vi "PreSequenceAcquisition.vi"(8 "error in (no error)":errorcluster, 11 "Camera_Prime95B in":refnum<class "Camera_Prime95B.lvclass">) -> (0 "error out":errorcluster, 3 "Camera_Prime95B out":refnum<class "Camera_Prime95B.lvclass">)   [LabVIEW 2020, in "Camera_Prime95B.lvlib" / "Camera_Prime95B.lvclass"]
uses:
  Camera_Prime95B.lvclass
  Hardware Abstraction Layer/Component/Device/Device/DataExchange.ctl
  Controls/AcquisitionParams.ctl
  Camera_Prime95B.lvclass/Camera_Prime95B.ctl
  E:/Development/DevHardSoftware/MicroscopyFramework/Model/Hardware Layer/Real Hardware/Camera_Prime95B/Camera_Prime95B/Dependencies/PVCamNET.dll
  Dependencies/PVCamNET.dll
  Interface/DataListener/DataListener.lvclass
panel:
  in  "DataExchange":T1
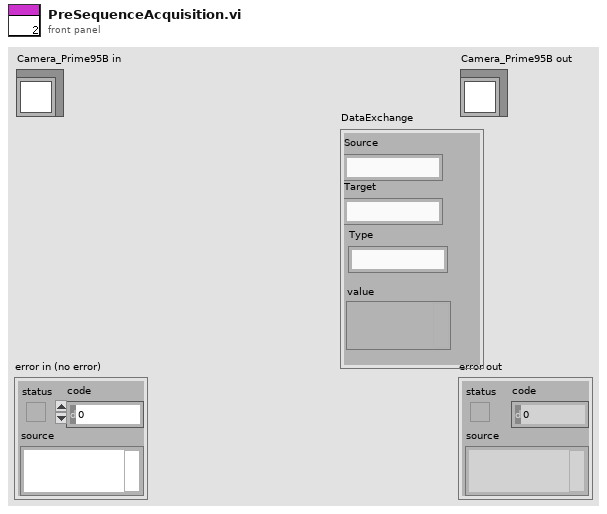
[diagram p1: front panel]
types:
  T1 = typedef "DataListener.lvclass/DataExchange.ctl" = cluster{"Source":string, "Target":string, "Type":string, "value":variant}
  T2 = typedef "Camera_Prime95B.lvlib/Camera_Prime95B.lvclass/AcquisitionParams.ctl" = cluster{"ExposureMs":dbl, "Frames":dbl, "Interval":dbl, "Save Path":path, "Stream Save Path":path, "SingleStack?":bool, "StreamToDisk?":bool, "Alert when finish?":bool, "File suffix":string, "Live?":bool}
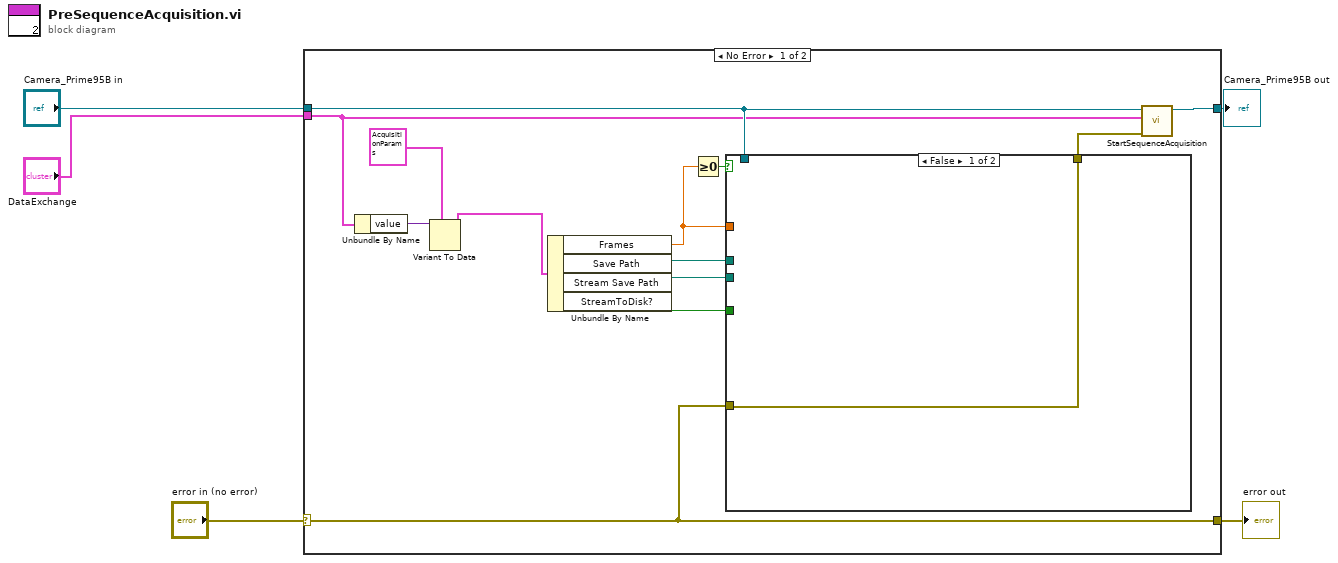
[diagram p0: block diagram]
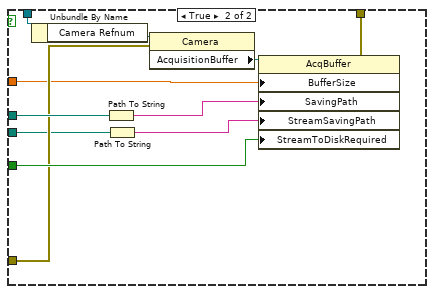
[diagram p2: hidden frame]
diagram:
  n1 = case shown="No Error" "error in (no error)" {
    selector: "error in (no error)" -> [w13 w32]
    tunnel: [w13 w32] -> w4
    tunnel: [w18 w31] -> w2
    tunnel: "Camera_Prime95B in" -> [w15 w31]
    tunnel: "DataExchange" -> [w8 _]
    frame No Error {
      n2 = Unbundle By Name(w8) -> ("value"=w9:variant)
      n3 = Variant To Data(type=T2 {"ExposureMs"=0.0, "Frames"=0.0, "Interval"=0.0, "Save Path"=path "", "Stream Save Path"=path "", "SingleStack?"=FALSE, "StreamToDisk?"=FALSE, "Alert when finish?"=FALSE, "File suffix"="", "Live?"=FALSE} ("Acquisition Params"), Variant=w9) -> (data=w7:T2)  [unwired: 1 in, 1 out]
      n4 = Unbundle By Name(w7) -> ("Frames"=w10:dbl, "Save Path"=w16:path, "Stream Save Path"=w11:path, "StreamToDisk?"=w12:bool)
      n5 = Greater Or Equal To 0?(x=w10) -> (x >= 0?=w17:bool)
      n6 = case shown="False" w17 {
        tunnel: w16 -> [_ w26]
        tunnel: w15 -> [_ w30]
        tunnel: w12 -> [_ w27]
        tunnel: [w19 w25] -> w14
        tunnel: w13 -> [w19 w24]
        tunnel: w11 -> [_ w23]
        tunnel: w10 -> [_ w20]
        frame False {
        }
        frame True {
          n7 = Unbundle By Name(w30) -> ("Camera Refnum"=w29:refnum<k24>)
          n8 = Path To String(path=w26) -> (string=w21:string)
          n9 = Path To String(path=w23) -> (string=w22:string)
          n10 = property class="Camera"(reference=w29, error in=w24) -> ("AcquisitionBuffer"=w28:refnum<k24>)  [unwired: 2 out]
          n11 = property class="AcqBuffer"(reference=w28, "BufferSize"=w20, "SavingPath"=w21, "StreamSavingPath"=w22, "StreamToDiskRequired"=w27) -> (error out=w25:errorcluster)  [unwired: 1 in, 1 out]
        }
      }
      n12 = call-dynamic "StartSequenceAcquisition.vi"("error in (no error)"=w14, "DataExchange"=w8, "Camera_Prime95B in"=w15) -> ("Camera_Prime95B out"=w18:refnum<class "Camera_Prime95B.lvclass">)  [unwired: 7 in, 1 out]
    }
    frame Error {
    }
  }
  "error out" <- w4
  "Camera_Prime95B out" <- w2
